vi "Index Path from Path.vi"(11 "Project Path":path) -> (3 "appended path":path)   [LabVIEW 2020, in "Test Finder.lvclass"]
uses:
  Test Finder.lvclass
  Test Finder.lvclass/Test Finder.ctl
  User Interface/Support/Paths.lvlib
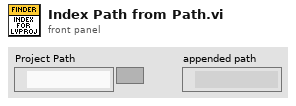
[diagram p1: front panel]
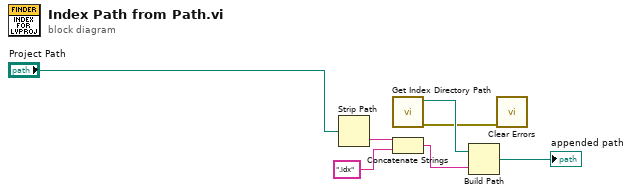
[diagram p0: block diagram]
diagram:
  n1 = Strip Path(path="Project Path") -> (name=w3:string)  [unwired: 1 out]
  n2 = call "Get Index Directory Path.vi"() -> ("error out"=w1:errorcluster, "Index Directory"=w5:path)  [unwired: 10 in]
  n3 = Concatenate Strings(w3, ".idx" ("string")) -> (w6:string)
  n4 = Build Path(base path=w5, name or relative path=w6) -> (appended path=→"appended path":path)
  n5 = call <vilib>:"Clear Errors.vi"("error in (no error)"=w1) -> ()  [unwired: 5 in, 2 out]
